vi "BCU诊断标定.vi"(8 "CAN端口":u16(ring), 9 "设备索引号":u16(ring), 10 "CAN卡类型":u32(ring)=21) -> ()   [LabVIEW 2013] (continued)
                                N: w5013 -> [_]
                                tunnel: [""] -> w5019 mode=indexing
                              }
                              n3537 = Multiply(x=u8 3, y=w5014) -> (x*y=w5016:dbl)
                              n3538 = Add(x=w5016, y=u8 23) -> (x+y=w5012:dbl)
                              n3539 = call "表格数据输入-8.6.vi"("行数"=w5012, "列数"=u32 1, "字符串数组"=w5019, "表格引用"=w5020) -> ()  [unwired: 8 in]
                            }
                            frame "保险位置" {
                              n3540 = local read "从板个数"() -> (w5024:dbl)
                              n3541 = control-ref of="项目信息"() -> (w5030:refnum<vi>)
                              n3542 = for {
                                N: 10 -> [_]
                                tunnel: [""] -> w5029 mode=indexing
                              }
                              n3543 = Multiply(x=u8 4, y=w5024) -> (x*y=w5026:dbl)
                              n3544 = Add(x=w5026, y=u8 24) -> (x+y=w5023:dbl)
                              n3545 = call "表格数据输入-8.6.vi"("行数"=w5023, "列数"=u32 1, "字符串数组"=w5029, "表格引用"=w5030) -> ()  [unwired: 8 in]
                            }
                            frame "电池额定实际容量" {
                              w5032 = 0.0 ("值")
                              n3546 = control-ref of="电池实际容量(A)"() -> (w5033:refnum<vi>)
                              n3547 = control-ref of="电池额定容量(A)"() -> (w5034:refnum<vi>)
                              n3548 = property class="DigNum (严格)"(reference=w5033, "Value"=w5032) -> ()  [unwired: 1 in, 2 out]
                              n3549 = property class="DigNum (严格)"(reference=w5034, "Value"=w5032) -> ()  [unwired: 1 in, 2 out]
                            }
                            frame "SOC" {
                              n3550 = control-ref of="SOC(%)"() -> (w5035:refnum<vi>)
                              n3551 = property class="DigNum (严格)"(reference=w5035, "Value"=0.0 ("值")) -> ()  [unwired: 1 in, 2 out]
                            }
                            frame "配置文件版本" {
                              n3552 = control-ref of="配置文件版本"() -> (w5037:refnum<vi>)
                              n3553 = property class="Str"(reference=w5037, "Value"="" ("值")) -> ()  [unwired: 1 in, 2 out]
                            }
                            frame "参数修改记录" {
                              n3554 = control-ref of="使用者"() -> (w5040:refnum<vi>)
                              n3555 = control-ref of="系统时钟"() -> (w5041:refnum<vi>)
                              n3556 = property class="DigNum (严格)"(reference=w5040, "Value"=0.0 ("值")) -> ()  [unwired: 1 in, 2 out]
                              n3557 = property class="Str"(reference=w5041, "Value"="" ("值")) -> ()  [unwired: 1 in, 2 out]
                            }
                            frame "校正时钟" {
                              n3558 = control-ref of="系统时钟"() -> (w5043:refnum<vi>)
                              n3559 = property class="Str"(reference=w5043, "Value"="" ("值")) -> ()  [unwired: 1 in, 2 out]
                            }
                            frame "车牌号" {
                              n3560 = control-ref of="车架(牌)号"() -> (w5045:refnum<vi>)
                              n3561 = property class="Str"(reference=w5045, "Value"="" ("值")) -> ()  [unwired: 1 in, 2 out]
                            }
                            frame "SOH" {
                              n3562 = control-ref of="SOH(%)"() -> (w5048:refnum<vi>)
                              n3563 = property class="DigNum (严格)"(reference=w5048, "Value"=0.0 ("值")) -> ()  [unwired: 1 in, 2 out]
                            }
                            frame "一级故障阀值" {
                              n3564 = local write "一级故障"(T10 {"总电压过高"=0.0, "整组电压不均衡"=0.0, "SOC过高"=0.0, "单体电压过高"=0.0, "总电压过低"=0.0, "温度过高"=0.0, "温度过低"=0.0, "单组电压不均衡"=0.0, "整组温度不均衡"=0.0, "单组温度不均衡"=0.0, "单体电压过低"=0.0, "充电电流过高"=0.0, "放电电流过高"=0.0, "SOC过低"=0.0, "内阻过大"=0.0, "极柱温度过高"=0.0, "SOH过低"=0.0} ("一级故障")) -> ()
                            }
                            frame "二级故障阀值" {
                              n3565 = local write "一级故障 2"(T10 {"总电压过高"=0.0, "整组电压不均衡"=0.0, "SOC过高"=0.0, "单体电压过高"=0.0, "总电压过低"=0.0, "温度过高"=0.0, "温度过低"=0.0, "单组电压不均衡"=0.0, "整组温度不均衡"=0.0, "单组温度不均衡"=0.0, "单体电压过低"=0.0, "充电电流过高"=0.0, "放电电流过高"=0.0, "SOC过低"=0.0, "内阻过大"=0.0, "极柱温度过高"=0.0, "SOH过低"=0.0} ("一级故障")) -> ()
                            }
                            frame "三级故障阀值" {
                              n3566 = local write "一级故障 3"(T10 {"总电压过高"=0.0, "整组电压不均衡"=0.0, "SOC过高"=0.0, "单体电压过高"=0.0, "总电压过低"=0.0, "温度过高"=0.0, "温度过低"=0.0, "单组电压不均衡"=0.0, "整组温度不均衡"=0.0, "单组温度不均衡"=0.0, "单体电压过低"=0.0, "充电电流过高"=0.0, "放电电流过高"=0.0, "SOC过低"=0.0, "内阻过大"=0.0, "极柱温度过高"=0.0, "SOH过低"=0.0} ("一级故障")) -> ()
                            }
                            frame "加热控制参数" {
                              n3567 = local write "加热控制参数"(T11 {"风机开启温度"=0.0, "风机关闭温度"=0.0, "加热开启温度"=0.0, "加热关闭温度"=0.0, "风机开启温差"=0.0, "风机关闭温差"=0.0, "加热关闭温差"=0.0} ("加热控制参数")) -> ()
                            }
                            frame "充电控制参数" {
                              n3568 = local write "一级故障 5"(T12 {"最大允许单体电压"=0.0, "最大允许总电压"=0.0, "最小允许单体电压"=0.0, "最大允许充电电流"=0.0, "最小允许充电电流"=0.0, "最大允许充电温度"=0.0, "最小允许充电温度"=0.0, "电流步长"=0.0} ("一级故障 5")) -> ()
                            }
                            frame "电池信息1" {
                              w5054 = ""
                              w5055 = 0.0 ("电池串联")
                              n3569 = local read "电池信息"() -> (w5057:T13)
                              n3570 = Bundle By Name(cluster=w5057, "电池串联"=w5055, "电池并联"=w5055, "电池包额定容量"=w5055, "电池包额定能量(kWh)"=w5055, "电池包额定总电压"=w5055, "实际容量"=w5055, "电池厂家"=w5054, "电池类型"=w5054, "电池生产日期"=w5054) -> (w5056:T13)
                              n3571 = local write "电池信息"(w5056) -> ()
                            }
                            frame "电池包组号" {
                              n3572 = local read "电池信息"() -> (w5060:T13)
                              n3573 = Bundle By Name(cluster=w5060, "电池包组号"="") -> (w5059:T13)
                              n3574 = local write "电池信息"(w5059) -> ()
                            }
                            frame "充放电安时" {
                              w5061 = 0.0 ("累计充电总安时")
                              n3575 = local read "电池信息"() -> (w5063:T13)
                              n3576 = Bundle By Name(cluster=w5063, "累计充电总安时"=w5061, "累计放电总安时"=w5061) -> (w5062:T13)
                              n3577 = local write "电池信息"(w5062) -> ()
                            }
                            frame "电池充放电次数" {
                              w5064 = 0.0 ("累计充电总安时")
                              n3578 = local read "电池信息"() -> (w5066:T13)
                              n3579 = Bundle By Name(cluster=w5066, "电池充满次数"=w5064, "电池放空次数"=w5064, "电池充电次数"=w5064) -> (w5065:T13)
                              n3580 = local write "电池信息"(w5065) -> ()
                            }
                          }
                        }
                        frame "从板" {
                          n3581 = case shown="\"加热控制参数\"" w5067 {
                            frame "假", Default {
                            }
                            frame "电压起始值" {
                              n3582 = control-ref of="项目信息 2"() -> (w5069:refnum<vi>)
                              n3583 = for {
                                N: 1 -> [_]
                                tunnel: [""] -> w5072 mode=indexing
                              }
                              n3584 = call "表格数据输入-8.6.vi"("行数"=u32 0, "列数"=u32 1, "字符串数组"=w5072, "表格引用"=w5069) -> ()  [unwired: 8 in]
                            }
                            frame "通道电压节数" {
                              n3585 = control-ref of="项目信息 2"() -> (w5074:refnum<vi>)
                              n3586 = for {
                                N: 5 -> [_]
                                tunnel: [""] -> w5078 mode=indexing
                              }
                              n3587 = call "表格数据输入-8.6.vi"("行数"=u32 22, "列数"=u32 1, "字符串数组"=w5078, "表格引用"=w5074) -> ()  [unwired: 8 in]
                            }
                            frame "保险位置" {
                              n3588 = control-ref of="项目信息 2"() -> (w5080:refnum<vi>)
                              n3589 = for {
                                N: 20 -> [_]
                                tunnel: [""] -> w5084 mode=indexing
                              }
                              n3590 = call "表格数据输入-8.6.vi"("行数"=u32 2, "列数"=u32 1, "字符串数组"=w5084, "表格引用"=w5080) -> ()  [unwired: 8 in]
                            }
                            frame "温度起始值" {
                              n3591 = control-ref of="项目信息 2"() -> (w5086:refnum<vi>)
                              n3592 = for {
                                N: 1 -> [_]
                                tunnel: [""] -> w5090 mode=indexing
                              }
                              n3593 = call "表格数据输入-8.6.vi"("行数"=u32 1, "列数"=u32 1, "字符串数组"=w5090, "表格引用"=w5086) -> ()  [unwired: 8 in]
                            }
                            frame "加热控制参数" {
                              n3594 = local write "加热控制参数"(T11 {"风机开启温度"=0.0, "风机关闭温度"=0.0, "加热开启温度"=0.0, "加热关闭温度"=0.0, "风机开启温差"=0.0, "风机关闭温差"=0.0, "加热关闭温差"=0.0} ("加热控制参数")) -> ()
                            }
                            frame "一级故障阀值" {
                              n3595 = local write "一级故障 6"(T15 {"电压过高"=0.0, "电压过低"=0.0, "温度过高"=0.0, "温度过低"=0.0, "电压不均衡(V)"=0.0, "温度不均衡"=0.0, "SOC过低"=0.0} ("一级故障 6")) -> ()
                            }
                            frame "二级故障阀值" {
                              n3596 = local write "一级故障 7"(T15 {"电压过高"=0.0, "电压过低"=0.0, "温度过高"=0.0, "温度过低"=0.0, "电压不均衡(V)"=0.0, "温度不均衡"=0.0, "SOC过低"=0.0} ("一级故障 7")) -> ()
                            }
                            frame "三级故障阀值" {
                              n3597 = local write "一级故障 8"(T15 {"电压过高"=0.0, "电压过低"=0.0, "温度过高"=0.0, "温度过低"=0.0, "电压不均衡(V)"=0.0, "温度不均衡"=0.0, "SOC过低"=0.0} ("一级故障 7")) -> ()
                            }
                            frame "均衡参数" {
                              n3598 = local write "均衡参数"(T17 {"充电结束电压(90%)"=0.0, "充电结束电压(91%)"=0.0, "充电结束电压(92%)"=0.0, "充电结束电压(93%)"=0.0, "充电结束电压(94%)"=0.0, "均衡计算-电压高阀值1级"=0.0, "均衡计算-电压高阀值2级"=0.0, "均衡计算-电压低阀值1级"=0.0, "均衡计算-电压低阀值2级"=0.0, "均衡计算-最低电压阀值"=0.0, "均衡停止-最低电压阀值"=0.0, "均衡计算-电压极差阀值"=0.0, "充电结束电压(95%)"=0.0, "充电结束电压(96%)"=0.0, "充电结束电压(97%)"=0.0, "充电结束电压(98%)"=0.0, "充电结束电压(99%)"=0.0, "充电结束电压(100%)"=0.0} ("均衡参数")) -> ()
                            }
                            frame "均衡阀值" {
                              w5097 = sgl 0.0 ("均衡计算-电压高阀值1级")
                              n3599 = local read "均衡参数"() -> (w5098:T17)
                              n3600 = Bundle By Name(cluster=w5098, "均衡计算-电压高阀值1级"=w5097, "均衡计算-电压高阀值2级"=w5097, "均衡计算-电压低阀值1级"=w5097, "均衡计算-电压低阀值2级"=w5097, "均衡计算-最低电压阀值"=w5097, "均衡停止-最低电压阀值"=w5097, "均衡计算-电压极差阀值"=w5097) -> (w5099:T17)
                              n3601 = local write "均衡参数"(w5099) -> ()
                            }
                            frame "充电结束电压" {
                              w5100 = sgl 0.0 ("均衡计算-电压高阀值1级")
                              n3602 = local read "均衡参数"() -> (w5101:T17)
                              n3603 = Bundle By Name(cluster=w5101, "充电结束电压(90%)"=w5100, "充电结束电压(91%)"=w5100, "充电结束电压(92%)"=w5100, "充电结束电压(93%)"=w5100, "充电结束电压(94%)"=w5100, "充电结束电压(95%)"=w5100, "充电结束电压(96%)"=w5100, "充电结束电压(97%)"=w5100, "充电结束电压(98%)"=w5100, "充电结束电压(99%)"=w5100, "充电结束电压(100%)"=w5100) -> (w5102:T17)
                              n3604 = local write "均衡参数"(w5102) -> ()
                            }
                          }
                        }
                      }
                    }
                    frame #1 {
                      w5103 = FALSE ("流控帧")
                      w5104 = TRUE ("流控帧 2")
                      n3605 = global write "EV05全局变量1.vi" "写入超时"(w5103) -> ()
                      n3606 = global write "EV05全局变量1.vi" "流控帧"(w5103) -> ()
                      n3607 = local write "写?"(w5103) -> ()
                      n3608 = call <vilib>:"Set Busy.vi"("disable click? (T)"=w5103) -> ()  [unwired: 3 in, 8 out]
                      n3609 = local write "消除"(w5104) -> ()
                      n3610 = local write "控制1"(w5104) -> ()
                      n3611 = global write "EV05全局变量1.vi" "流控帧 2"(w5104) -> ()
                    }
                    frame #2 {
                      n3612 = Wait Until Next ms Multiple(millisecond multiple=u32 150 ("毫秒倍数")) -> ()  [unwired: 1 out]
                    }
                    frame #3 {
                      n3613 = local read "设备索引号"() -> (w5111:u16)
                      n3614 = local read "CAN卡类型"() -> (w5112:u32)
                      n3615 = local read "CAN端口"() -> (w5110:u16)
                      n3616 = stacked-sequence {
                        tunnel: w5112 -> [_ w5120]
                        tunnel: w5111 -> [_ w5119]
                        tunnel: w5110 -> [_ w5118]
                        tunnel: w5109 -> [_ w5117]
                        tunnel: w5108 -> [_ w5116]
                        tunnel: w5107 -> [_ w5115]
                        tunnel: w5106 -> [_ w5114]
                        frame #0 {
                        }
                        frame #1 {
                          n3617 = call "多帧发送机制(EV05).vi"("can卡类型"=w5120, "设备索引号"=w5119, "CAN端口"=w5118, "命令"=w5116, "板号"=w5115, "命令序号"=w5117, "输入数据"=w5114) -> ("错误输出"=w5113:errorcluster)  [unwired: 1 in, 11 out]
                          n3618 = call <vilib>:"Clear Errors.vi"("error in (no error)"=w5113) -> ()  [unwired: 6 in, 1 out]
                        }
                      }
                      "命令序号" <- w5109
                    }
                    frame #4 {
                      n3619 = while {
                        tunnel: [w5125] -> w5122
                        tunnel: [w5124] -> w5121
                        i -> [w5128]
                        stop <- w5125 stop-if-true
                        n3620 = local read "强制终止读写标记"() -> (w5123:bool)
                        n3621 = global read "EV05全局变量1.vi" "写入超时"() -> (w5124:bool)
                        n3622 = Greater Or Equal?(x=w5128, y=30) -> (x >= y?=w5126:bool)
                        n3623 = Compound Arithmetic op=OR(w5123, w5124, w5126) -> (w5125:bool)
                        n3624 = Wait Until Next ms Multiple(millisecond multiple=u32 100 ("毫秒倍数")) -> ()  [unwired: 1 out]
                      }
                    }
                    frame #5 {
                      n3625 = call <vilib>:"Unset Busy.vi"() -> ()  [unwired: 11 in, 1 out]
                      n3626 = case shown="假" w5130 {
                        tunnel: w5131 -> [w5134 _]
                        frame False {
                          n3627 = control-ref of="结果"() -> (w5133:refnum<vi>)
                          n3628 = Concatenate Strings(w5134, "     读取失败" ("字符串")) -> (w5136:string)
                          n3629 = Build Array(w5136) -> (w5132:string[])
                          n3630 = call "表格编辑.vi"("新元素/子数组"=w5132, "活动单元格:单元格背景色"=u32 16740749, "MCListbox引用句柄"=w5133) -> ()  [unwired: 9 out]
                        }
                        frame True {
                        }
                      }
                    }
                    frame #6 {
                      n3631 = Increment(x=w5140) -> (x+1=w5139:i32)
                      n3632 = Equal?(x=w5141, y=w5139) -> (x = y?=w5138:bool)
                      n3633 = case shown="真" w5138 {
                        frame False {
                        }
                        frame True {
                          n3634 = control-ref of="结果"() -> (w5143:refnum<vi>)
                          n3635 = Concatenate Strings("读取完成" ("字符串")) -> (w5145:string)
                          n3636 = Build Array(w5145) -> (w5142:string[])
                          n3637 = call "表格编辑.vi"("新元素/子数组"=w5142, "活动单元格:单元格背景色"=u32 21937, "MCListbox引用句柄"=w5143) -> ()  [unwired: 9 out]
                        }
                      }
                    }
                  }
                }
              }
            }
          }
          n3638 = stacked-sequence {
            tunnel: w4795 -> [_]
            frame #0 {
              n3639 = call <vilib>:"Unset Busy.vi"() -> ()  [unwired: 11 in, 1 out]
              n3640 = local write "强制终止读写标记"(FALSE ("强制停止")) -> ()
            }
          }
        }
        frame "全部读取" {
          n3641 = stacked-sequence {
            seq-local: [w5151 _ _] -> [_ _ w5706]
            seq-local: [w5150 _ _] -> [_ _ w5705]
            tunnel: [_ w5342 _] -> w5148
            frame #0 {
              n3642 = local read "主从选择"() -> (w5151:enum32{"主板", "从板"})
              n3643 = local read "路径"() -> (w5152:path)
              n3644 = Empty String/Path?(string/path=w5152) -> (empty?=w5150:bool)
              n3645 = disable-structure shown="禁用" {
                disable-tunnel: w5152 -> [w5155 _]
                disable-tunnel: w5150 -> [w5154 _]
                disable-tunnel: w5151 -> [w5153 _]
                frame Disabled {
                  n3646 = case shown="假" w5154 {
                    tunnel: w5155 -> [w5159 _]
                    tunnel: w5153 -> [w5158 _]
                    frame False {
                      n3647 = control-ref of="结果"() -> (w5156:refnum<vi>)
                      n3648 = call-poly <vilib>:"Read From Spreadsheet File.vi"("file path (dialog if empty)"=w5159) -> ("all rows"=w5157:string[][])  [unwired: 3 in, 7 out]
                      n3649 = case shown="\"主板\", 默认" w5158 {
                        tunnel: w5157 -> [w5161 w5256]
                        tunnel: w5156 -> [w5160 w5255]
                        frame "主板", Default {
                          n3650 = stacked-sequence {
                            tunnel: w5161 -> [w5170 w5194 w5251]
                            tunnel: w5160 -> [w5167 _ w5222]
                            frame #0 {
                              n3651 = Index Array(array=w5170, index (col)=3 ("禁用的索引 (列)")) -> (element=w5184:string[])  [unwired: 1 in]
                              n3652 = Index Array(array=w5170, index (col)=1 ("禁用的索引 (列)")) -> (element=w5190:string[])  [unwired: 1 in]
                              n3653 = Delete From Array(array=w5184, length=4 ("长度"), index=0 ("索引")) -> (deleted portion=w5181:string[], array with subset deleted=w5175:string[])
                              n3654 = Delete From Array(array=w5190, length=1 ("长度"), index=0 ("索引")) -> (deleted portion=w5187:string[], array with subset deleted=w5164:string[])
                              n3655 = Build Array("正在读取主板配置文件...") -> (w5168:string[])
                              n3656 = Index Array(array=w5175) -> (element #1=w5174:string, element #2=w5173:string, element #3=w5172:string, element #4=w5171:string)  [unwired: 4 in]
                              n3657 = for {
                                tunnel: w5181 -> [w5193] mode=indexing
                                tunnel: [w5192] -> w5180 mode=indexing
                                n3658 = Fract/Exp String To Number(string=w5193) -> (number=w5192:dbl)  [unwired: 4 out]
                              }
                              n3659 = Index Array(array=w5187) -> (element=w5186:string)  [unwired: 1 in]
                              n3660 = global write "读配置文件全局.vi" "表格输入"(w5164) -> ()
                              n3661 = call "表格编辑.vi"("新元素/子数组"=w5168, "活动单元格:单元格背景色"=u32 6618880, "MCListbox引用句柄"=w5167) -> ()  [unwired: 9 out]
                              n3662 = Decimal String To Number(string=w5186) -> (number=w5165:i32)  [unwired: 1 in, 2 out]
                              n3663 = global read "读配置文件全局.vi" "项目信息"() -> (w5163:T27)
                              n3664 = Index Array(array=w5180) -> (element #1=w5179:dbl, element #2=w5178:dbl, element #3=w5177:dbl, element #4=w5176:dbl)  [unwired: 4 in]
                              n3665 = global write "读配置文件全局.vi" "从板个数"(w5165) -> ()
                              n3666 = Bundle(cluster=w5163, "电池额定容量"=w5179, "电池实际容量"=w5178, "车牌号"=w5174, "配置文件版本"=w5173, "SOH"=w5176, "SOC"=w5177, "产品编号"=w5172, "系统时钟"=w5171) -> (w5162:T27)  [unwired: 1 out]
                              n3667 = global write "读配置文件全局.vi" "项目信息"(w5162) -> ()
                            }
                            frame #1 {
                              n3668 = Index Array(array=w5194, index (col)=3 ("禁用的索引 (列)")) -> (element=w5212:string[])  [unwired: 1 in]
                              n3669 = Index Array(array=w5194, index (col)=5 ("禁用的索引 (列)")) -> (element=w5206:string[])  [unwired: 1 in]
                              n3670 = for {
                                tunnel: w5206 -> [w5219] mode=indexing
                                tunnel: [w5218] -> w5205 mode=indexing
                                n3671 = Fract/Exp String To Number(string=w5219) -> (number=w5218:dbl)  [unwired: 4 out]
                              }
                              n3672 = Delete From Array(array=w5212, length=17 ("长度"), index=8 ("索引")) -> (deleted portion=w5210:string[])  [unwired: 1 out]
                              n3673 = for {
                                tunnel: w5210 -> [w5221] mode=indexing
                                tunnel: [w5220] -> w5208 mode=indexing
                                n3674 = Fract/Exp String To Number(string=w5221) -> (number=w5220:dbl)  [unwired: 4 out]
                              }
                              n3675 = global write "读配置文件全局.vi" "二级故障"(w5205) -> ()
                              n3676 = global write "读配置文件全局.vi" "一级故障"(w5208) -> ()
                              n3677 = Index Array(array=w5194, index (col)=7 ("禁用的索引 (列)")) -> (element=w5203:string[])  [unwired: 1 in]
                              n3678 = Index Array(array=w5194, index (col)=9 ("禁用的索引 (列)")) -> (element=w5200:string[])  [unwired: 1 in]
                              n3679 = for {
                                tunnel: w5203 -> [w5217] mode=indexing
                                tunnel: [w5216] -> w5202 mode=indexing
                                n3680 = Fract/Exp String To Number(string=w5217) -> (number=w5216:dbl)  [unwired: 4 out]
                              }
                              n3681 = for {
                                tunnel: w5200 -> [w5215] mode=indexing
                                tunnel: [w5214] -> w5199 mode=indexing
                                n3682 = Fract/Exp String To Number(string=w5215) -> (number=w5214:dbl)  [unwired: 4 out]
                              }
                              n3683 = Delete From Array(array=w5199, length=6 ("长度"), index=0 ("索引")) -> (deleted portion=w5196:dbl[], array with subset deleted=w5195:dbl[])
                              n3684 = global write "读配置文件全局.vi" "三级故障"(w5202) -> ()
                              n3685 = global write "读配置文件全局.vi" "加热控制参数"(w5196) -> ()
                              n3686 = global write "读配置文件全局.vi" "充电控制参数"(w5195) -> ()
                            }
                            frame #2 {
                              n3687 = call <vilib>:"Unset Busy.vi"() -> ()  [unwired: 2 in, 10 out]
                              n3688 = Index Array(array=w5251, index (col)=11 ("禁用的索引 (列)")) -> (element=w5248:string[])  [unwired: 1 in]
                              n3689 = Delete From Array(array=w5248, length=6 ("长度"), index=0 ("索引")) -> (deleted portion=w5230:string[], array with subset deleted=w5229:string[])
                              n3690 = for {
                                tunnel: w5229 -> [w5254] mode=indexing
                                tunnel: [w5253] -> w5247 mode=indexing
                                n3691 = Fract/Exp String To Number(string=w5254) -> (number=w5253:dbl)  [unwired: 4 out]
                              }
                              n3692 = Index Array(array=w5230) -> (element #1=w5246:string, element #2=w5245:string, element #3=w5244:string, element #4=w5243:string, element #5=w5242:string, element #6=w5241:string)  [unwired: 6 in]
                              n3693 = Index Array(array=w5247) -> (element #1=w5240:dbl, element #2=w5239:dbl, element #3=w5238:dbl, element #4=w5237:dbl, element #5=w5236:dbl, element #6=w5235:dbl, element #7=w5234:dbl, element #8=w5233:dbl, element #9=w5232:dbl, element #10=w5231:dbl, element #11=w5226:dbl)  [unwired: 11 in]
                              n3694 = global read "读配置文件全局.vi" "电池信息"() -> (w5228:T28)
                              n3695 = Build Array("配置文件读取完成") -> (w5224:string[])
                              n3696 = Bundle(cluster=w5228, "电池串联"=w5240, "电池并联"=w5239, "累计放电总安时"=w5237, "电池包额定容量"=w5236, "电池包额定能量"=w5235, "电池包额定总电压"=w5234, "累计充电总安时"=w5238, "电池充满次数"=w5233, "电池放空次数"=w5232, "电池充电次数"=w5231, "电池生产日期"=w5246, "电池厂家"=w5245, "电池类型"=w5244, "电池包组号"=w5243, "电池包产权标识"=w5242, "电池应用车型"=w5241, "实际容量"=w5226) -> (w5227:T28)
                              n3697 = call "表格编辑.vi"("新元素/子数组"=w5224, "活动单元格:单元格背景色"=u32 6618880, "MCListbox引用句柄"=w5222) -> ()  [unwired: 9 out]
                              n3698 = global write "读配置文件全局.vi" "电池信息"(w5227) -> ()
                            }
                          }
                        }
                        frame "从板" {
                          n3699 = stacked-sequence {
                            tunnel: w5256 -> [w5264 w5292 w5336]
                            tunnel: w5255 -> [w5261 _ w5312]
                            frame #0 {
                              n3700 = Index Array(array=w5264, index (col)=1 ("禁用的索引 (列)")) -> (element=w5274:string[])  [unwired: 1 in]
                              n3701 = Index Array(array=w5264, index (col)=3 ("禁用的索引 (列)")) -> (element=w5268:string[])  [unwired: 1 in]
                              n3702 = Delete From Array(array=w5274, length=1 ("长度"), index=0 ("索引")) -> (deleted portion=w5271:string[], array with subset deleted=w5258:string[])
                              n3703 = Delete From Array(array=w5268, length=6 ("长度"), index=0 ("索引")) -> (deleted portion=w5265:string[])  [unwired: 1 out]
                              n3704 = for {
                                tunnel: w5265 -> [w5277] mode=indexing
                                tunnel: [w5276] -> w5257 mode=indexing
                                i -> [w5278]
                                n3705 = Fract/Exp String To Number(string=w5277, default (0 dbl)=w5278) -> (number=w5276:i32)  [unwired: 3 out]
                              }
                              n3706 = Index Array(array=w5271) -> (element=w5270:string)  [unwired: 1 in]
                              n3707 = global write "读配置文件全局2.vi" "表格"(w5258) -> ()
                              n3708 = Build Array("正在读取从板配置文件...") -> (w5262:string[])
                              n3709 = Decimal String To Number(string=w5270) -> (number=w5259:i32)  [unwired: 1 in, 2 out]
                              n3710 = call "表格编辑.vi"("新元素/子数组"=w5262, "活动单元格:单元格背景色"=u32 6618880, "MCListbox引用句柄"=w5261) -> ()  [unwired: 9 out]
                              n3711 = global write "读配置文件全局2.vi" "加热控制参数"(w5257) -> ()
                              n3712 = global write "读配置文件全局2.vi" "从板板号"(w5259) -> ()
                            }
                            frame #1 {
                              n3713 = Index Array(array=w5292, index (col)=3 ("禁用的索引 (列)")) -> (element=w5282:string[])  [unwired: 1 in]
                              n3714 = Array Subset(array=w5282, index=6 ("索引"), length=7 ("长度")) -> (w5289:string[])
                              n3715 = Array Subset(array=w5282, index=13 ("索引"), length=7 ("长度")) -> (w5288:string[])
                              n3716 = Array Subset(array=w5282, index=20 ("索引"), length=7 ("长度")) -> (w5283:string[])
                              n3717 = for {
                                tunnel: w5289 -> [w5299] mode=indexing
                                tunnel: [w5298] -> w5279 mode=indexing
                                n3718 = Fract/Exp String To Number(string=w5299) -> (number=w5298:dbl)  [unwired: 4 out]
                              }
                              n3719 = for {
                                tunnel: w5288 -> [w5297] mode=indexing
                                tunnel: [w5296] -> w5280 mode=indexing
                                n3720 = Fract/Exp String To Number(string=w5297) -> (number=w5296:dbl)  [unwired: 4 out]
                              }
                              n3721 = for {
                                tunnel: w5283 -> [w5295] mode=indexing
                                tunnel: [w5294] -> w5281 mode=indexing
                                n3722 = Fract/Exp String To Number(string=w5295) -> (number=w5294:dbl)  [unwired: 4 out]
                              }
                              n3723 = global write "读配置文件全局2.vi" "一级故障阀值"(w5279) -> ()
                              n3724 = global write "读配置文件全局2.vi" "二级故障阀值"(w5280) -> ()
                              n3725 = global write "读配置文件全局2.vi" "三级故障阀值"(w5281) -> ()
                            }
                            frame #2 {
                              n3726 = Index Array(array=w5336, index (col)=5 ("禁用的索引 (列)")) -> (element=w5334:string[])  [unwired: 1 in]
                              n3727 = Delete From Array(array=w5334, length=1 ("长度"), index=16 ("索引")) -> (deleted portion=w5330:string[], array with subset deleted=w5331:string[])
                              n3728 = for {
                                tunnel: w5331 -> [w5339] mode=indexing
                                tunnel: [w5338] -> w5335 mode=indexing
                                n3729 = Fract/Exp String To Number(string=w5339) -> (number=w5338:dbl)  [unwired: 4 out]
                              }
                              n3730 = Index Array(array=w5335) -> (element #1=w5329:dbl, element #2=w5328:dbl, element #3=w5327:dbl, element #4=w5326:dbl, element #5=w5325:dbl, element #6=w5324:dbl, element #7=w5323:dbl, element #8=w5322:dbl, element #9=w5321:dbl, element #10=w5320:dbl, element #11=w5319:dbl, element #12=w5310:dbl, element #13=w5318:dbl, element #14=w5317:dbl, element #15=w5316:dbl, element #16=w5315:dbl, element #17=w5308:dbl, element #18=w5307:dbl, element #19=w5306:dbl, element #20=w5305:dbl, element #21=w5304:dbl, element #22=w5303:dbl)  [unwired: 22 in]
                              n3731 = Build Array("配置文件读取完成") -> (w5313:string[])
                              n3732 = Index Array(array=w5330, index=22 ("索引")) -> (element=w5309:string)
                              n3733 = global read "读配置文件全局2.vi" "电池组信息"() -> (w5301:T29)
                              n3734 = call "表格编辑.vi"("新元素/子数组"=w5313, "活动单元格:单元格背景色"=u32 6618880, "MCListbox引用句柄"=w5312) -> ()  [unwired: 9 out]
                              n3735 = Bundle(cluster=w5301, "电池类型"=w5329, "电池厂家"=w5328, "电池地区"=w5327, "电池组序号"=w5326, "电池包串联数"=w5325, "电池包并联数"=w5324, "电池包安时数"=w5323, "电池包序号"=w5322, "充电次数"=w5321, "充满电时间"=w5320, "放空时间"=w5319, "车牌号"=w5309, "最大允许单体电压"=w5310, "最大允许总电压"=w5318, "最大允许温度"=w5317, "最小允许温度"=w5316, "最大允许充电电流"=w5315, "最小允许充电电流"=w5308, "最小允许单体电压"=w5307, "电流步长"=w5306, "SOC"=w5305, "充电总安时"=w5304, "放电总这时"=w5303) -> (w5300:T29)
                              n3736 = call <vilib>:"Unset Busy.vi"() -> ()  [unwired: 2 in, 10 out]
                              n3737 = global write "读配置文件全局2.vi" "电池组信息"(w5300) -> ()
                            }
                          }
                        }
                      }
                    }
                    frame True {
                    }
                  }
                }
                frame Enabled {
                }
              }
              n3738 = case shown="\"从板\"" w5151 {
                frame "主板", Default {
                  w5340 = FALSE
                  n3739 = global write "读配置文件全局.vi" "SOC判定"(w5340) -> ()
                  n3740 = global write "读配置文件全局.vi" "SOH判定"(w5340) -> ()
                  n3741 = global write "读配置文件全局.vi" "车牌号判定"(w5340) -> ()
                  n3742 = global write "读配置文件全局.vi" "电池信息1判定"(w5340) -> ()
                  n3743 = global write "读配置文件全局.vi" "保险位置判定"(w5340) -> ()
                  n3744 = global write "读配置文件全局.vi" "产品编号判定"(w5340) -> ()
                  n3745 = global write "读配置文件全局.vi" "充放电安时判定"(w5340) -> ()
                  n3746 = global write "读配置文件全局.vi" "从板个数判定"(w5340) -> ()
                  n3747 = global write "读配置文件全局.vi" "电池包组号判定"(w5340) -> ()
                  n3748 = global write "读配置文件全局.vi" "电压个数判定"(w5340) -> ()
                  n3749 = global write "读配置文件全局.vi" "电压起始值判定"(w5340) -> ()
                  n3750 = global write "读配置文件全局.vi" "二级故障判定"(w5340) -> ()
                  n3751 = global write "读配置文件全局.vi" "三级故障判定"(w5340) -> ()
                  n3752 = global write "读配置文件全局.vi" "通道电压数判定"(w5340) -> ()
                  n3753 = global write "读配置文件全局.vi" "温度个数判定"(w5340) -> ()
                  n3754 = global write "读配置文件全局.vi" "一级故障判定"(w5340) -> ()
                  n3755 = global write "读配置文件全局.vi" "温度起始值判定"(w5340) -> ()
                  n3756 = global write "读配置文件全局.vi" "充电控制参数判定"(w5340) -> ()
                  n3757 = global write "读配置文件全局.vi" "电池充放电次数判定"(w5340) -> ()
                  n3758 = global write "读配置文件全局.vi" "加热控制参数判定"(w5340) -> ()
                  n3759 = global write "读配置文件全局.vi" "配置文件版本判定"(w5340) -> ()
                  n3760 = global write "读配置文件全局.vi" "电池额定实际容量判定"(w5340) -> ()
                }
                frame "从板" {
                  w5341 = FALSE
                  n3761 = disable-structure shown="禁用" {
                    frame Disabled {
                      n3762 = global read "读配置文件全局2.vi" "充电次数时间判定"() -> ()  [unwired: 1 in]
                      n3763 = global read "读配置文件全局2.vi" "电池包信息1判定"() -> ()  [unwired: 1 in]
                      n3764 = global read "读配置文件全局2.vi" "电池包序号判定"() -> ()  [unwired: 1 in]
                      n3765 = global read "读配置文件全局2.vi" "充放电安时判定"() -> ()  [unwired: 1 in]
                      n3766 = global read "读配置文件全局2.vi" "车牌号判定"() -> ()  [unwired: 1 in]
                      n3767 = global read "读配置文件全局2.vi" "充电参数判定"() -> ()  [unwired: 1 in]
                      n3768 = global read "读配置文件全局2.vi" "保险位置判定"() -> ()  [unwired: 1 in]
                    }
                    frame Enabled {
                    }
                  }
                  n3769 = global write "读配置文件全局2.vi" "从板号判定"(w5341) -> ()
                  n3770 = global write "读配置文件全局2.vi" "通道电压判定"(w5341) -> ()
                  n3771 = global write "读配置文件全局2.vi" "保险位置判定"(w5341) -> ()
                  n3772 = global write "读配置文件全局2.vi" "二级故障判定"(w5341) -> ()
                  n3773 = global write "读配置文件全局2.vi" "三级故障判定"(w5341) -> ()
                  n3774 = global write "读配置文件全局2.vi" "一级故障判定"(w5341) -> ()
                  n3775 = global write "读配置文件全局2.vi" "电压起始值判定"(w5341) -> ()
                  n3776 = global write "读配置文件全局2.vi" "温度起始值判定"(w5341) -> ()
                }
              }
            }
            frame #1 {
              (unwired) "均衡参数"
              # "去掉加热控制信息 20140106"
              n3777 = local read "主从选择"() -> (w5345:enum32{"主板", "从板"})
              n3778 = case shown="\"主板\", 默认" w5345 {
                tunnel: [string[] ["项目信息", "一级故障阀值", "二级故障阀值", "三级故障阀值", "加热控制信息", "充电控制信息", "电池信息"] string[] ["从板信息", "一级故障阀值", "二级故障阀值", "三级故障阀值"]] -> w5344
                frame "主板", Default {
                }
                frame "从板" {
                }
              }
              n3779 = Array Size(array=w5344) -> (size(s)=w5343:i32)
              n3780 = for {
                tunnel: w5344 -> [w5361] mode=indexing
                tunnel: w5345 -> [w5349]
                tunnel: w5343 -> [w5353]
                tunnel: [w5348] -> w5342
                i -> [w5350]
                n3781 = case shown="\"主板\", 默认" w5349 {
                  tunnel: [w5657 w5685] -> w5355
                  tunnel: [w5656 w5686] -> w5356
                  tunnel: w5361 -> [w5653 w5682]
                  tunnel: [u8 0 ("板号") w5683] -> w5360
                  tunnel: [u8 0 ("板号") u8 0 ("板号")] -> w5359
                  tunnel: [w5652 w5681] -> w5357
                  frame "主板", Default {
                    n3782 = case shown="\"项目信息\"" w5653 {
                      tunnel: [_ u8[] [1, 2, 3, 4, 5, 6, 13, 8, 7, 9, 10, 11, 12] u8[] [1] u8[] [2] u8[] [3] u8[] [1] u8[] [2] u8[] [1, 2, 3] u8[] [1, 2, 3, 4]] -> w5657
                      tunnel: [_ u8 128 ("命令") u8 129 ("命令") u8 129 ("命令") u8 129 ("命令") u8 130 ("命令") u8 130 ("命令") u8 131 ("命令") u8 132 ("命令")] -> w5656
                      tunnel: [_ string[] ["产品编号", "电压个数", "通道电压数", "电压起始值", "温度个数", "温度起始值", "保险位置", "电池额定实际容量", "SOC", "配置文件版本", "参数修改记录", "车牌号", "SOH"] string[] ["一级故障阀值"] string[] ["二级故障阀值"] string[] ["三级故障阀值"] string[] ["加热控制参数"] string[] ["充电控制参数"] _ string[] ["电池信息1", "电池包组号", "充放电安时", "电池充放电次数"]] -> w5652
                      frame "假", Default {
                      }
                      frame "项目信息" {
                      }
                      frame "一级故障阀值" {
                      }
                      frame "二级故障阀值" {
                      }
                      frame "三级故障阀值" {
                      }
                      frame "加热控制信息" {
                      }
                      frame "充电控制信息" {
                      }
                      frame "历史信息" {
                      }
                      frame "电池信息" {
                      }
                    }
                  }
                  frame "从板" {
                    n3783 = case shown="\"从板信息\"" w5682 {
                      tunnel: [_ u8 0 ("命令") u8 2 ("命令") u8 2 ("命令") u8 2 ("命令") u8 3 ("命令") u8 6 ("命令")] -> w5686
                      tunnel: [_ u8[] [6, 1, 2, 3, 4, 5] u8[] [1] u8[] [2] u8[] [3] u8[] [1, 2, 3, 4, 5, 6, 7] u8[] [1, 2]] -> w5685
                      tunnel: [_ string[] ["从板号", "电压起始值", "通道电压节数", "保险位置", "温度起始值", "加热控制参数"] string[] ["一级故障阀值"] string[] ["二级故障阀值"] string[] ["三级故障阀值"] string[] ["电池包信息1", "电池包序号", "充放电安时", "充电次数时间", "SOC", "车牌号", "充电参数"] string[] ["均衡阀值", "充电结束电压"]] -> w5681
                      frame "假", Default {
                      }
                      frame "从板信息" {
                      }
                      frame "一级故障阀值" {
                      }
                      frame "二级故障阀值" {
                      }
                      frame "三级故障阀值" {
                      }
                      frame "快换参数" {
                      }
                      frame "均衡参数" {
                      }
                    }
                    n3784 = local read "从板号"() -> (w5683:u8)
                  }
                }
                n3785 = Increment(x=w5350) -> (x+1=w5352:i32)
                n3786 = Equal?(x=w5353, y=w5352) -> (x = y?=w5351:bool)
                n3787 = case shown="\"从板\"" w5349 {
                  tunnel: w5350 -> [w5623 w5637]
                  frame "主板", Default {
                    n3788 = case shown="0, 默认" w5623 {
                      tunnel: [T8."项目信息" ("主从板") T8."一级故障阀值" ("主从板") T8."二级故障阀值" ("主从板") T8."三级故障阀值" ("主从板") T8."控制参数" ("主从板") T8."电池信息" ("主从板")] -> w5622
                      frame 0, Default {
                        n3789 = local write "1"(TRUE ("1")) -> ()
                      }
                      frame 1 {
                        n3790 = local write "1 2"(TRUE ("1 2")) -> ()
                      }
                      frame 2 {
                        n3791 = local write "1 3"(TRUE ("1 3")) -> ()
                      }
                      frame 3 {
                        n3792 = local write "1 4"(TRUE ("1 4")) -> ()
                      }
                      frame 4, 5 {
                        n3793 = local write "1 5"(TRUE ("1 5")) -> ()
                      }
                      frame 6 {
                        n3794 = local write "1 11"(TRUE ("1 11")) -> ()
                      }
                    }
                    n3795 = local write "主板2"(w5622) -> ()
                  }
                  frame "从板" {
                    n3796 = case shown="4" w5637 {
                      tunnel: [T21."从板信息" ("等级 2") T21."从板信息" ("等级 2") T21."一级故障阀值" ("等级 2") T21."二级故障阀值" ("等级 2") T21."三级故障阀值" ("等级 2") T21."快换参数" ("等级 2") T14."均衡参数" ("等级 2")] -> w5636
                      frame 99, Default {
                        n3797 = local write "1 6"(TRUE ("1 6")) -> ()
                      }
                      frame 0 {
                        n3798 = local write "1 6"(TRUE ("1 6")) -> ()
                      }
                      frame 1 {
                        n3799 = local write "1 7"(TRUE ("1 7")) -> ()
                      }
                      frame 2 {
                        n3800 = local write "1 8"(TRUE ("1 8")) -> ()
                      }
                      frame 3 {
                        n3801 = local write "1 9"(TRUE ("1 9")) -> ()
                      }
                      frame 5 {
                        n3802 = local write "1 10"(TRUE ("1 10")) -> ()
                      }
                      frame 4 {
                        n3803 = local write "1 12"(TRUE ("1 10")) -> ()
                      }
                    }
                    n3804 = local write "等级 2"(w5636) -> ()
                  }
                }
                n3805 = Array Size(array=w5355) -> (size(s)=w5354:i32)
                n3806 = local write "命令"(w5356) -> ()
                n3807 = Build Array(w5359) -> (w5358:u8[])
                n3808 = while {
                  tunnel: w5356 -> [w5393]
                  tunnel: w5360 -> [w5392]
                  tunnel: w5358 -> [w5391]
                  tunnel: w5354 -> [w5387]
                  tunnel: w5351 -> [w5390]
                  tunnel: w5349 -> [w5384]
                  tunnel: [w5383] -> w5348
                  shift-right: [w5382] -> _
                  shift-left: w5357 -> [w5363]
                  shift-right: [w5373] -> _
                  shift-left: w5355 -> [w5362]
                  i -> [w5388]
                  stop <- w5383 stop-if-true
                  n3809 = local read "强制终止读写标记"() -> (w5379:bool)
                  n3810 = Array Size(array=w5363) -> (size(s)=w5381:i32)
                  n3811 = Increment(x=w5388) -> (x+1=w5389:i32)
                  n3812 = Greater Than 0?(x=w5381) -> (x > 0?=w5380:bool)
                  n3813 = Equal?(x=w5387, y=w5389) -> (x = y?=w5385:bool)
                  n3814 = Not(x=w5379) -> (.not. x?=w5378:bool)
                  n3815 = And(x=w5378, y=w5380) -> (x .and. y?=w5377:bool)
                  n3816 = Delete From Array(array=w5363, length=1 ("长度"), index=0 ("索引")) -> (deleted portion=w5369:string[], array with subset deleted=w5374:string[])
                  n3817 = Index Array(array=w5369, index=0 ("索引")) -> (element=w5367:string)
                  n3818 = Delete From Array(array=w5362, length=1 ("长度"), index=0 ("索引")) -> (deleted portion=w5365:u8[], array with subset deleted=w5370:u8[])
                  n3819 = Index Array(array=w5365, index=0 ("索引")) -> (element=w5364:u8)
                  n3820 = case shown="真" w5377 {
                    tunnel: w5393 -> [_ w5409]
                    tunnel: w5364 -> [_ w5408]
                    tunnel: w5392 -> [_ w5407]
                    tunnel: w5391 -> [_ w5406]
                    tunnel: w5367 -> [_ w5405]
                    tunnel: w5390 -> [_ w5404]
                    tunnel: w5385 -> [_ w5403]
                    tunnel: w5384 -> [_ w5402]
                    tunnel: [string[] [] w5398] -> w5382
                    tunnel: w5374 -> [_ w5401]
                    tunnel: [u8[] [] w5396] -> w5373
                    tunnel: w5370 -> [_ w5400]
                    tunnel: w5363 -> [_ w5399]
                    tunnel: w5362 -> [_ w5397]
                    frame False {
                    }
                    frame True {
                      n3821 = while {
                        tunnel: w5409 -> [w5425]
                        tunnel: w5408 -> [w5424]
                        tunnel: w5407 -> [w5423]
                        tunnel: w5406 -> [w5422]
                        tunnel: w5405 -> [w5420]
                        tunnel: w5404 -> [w5419]
                        tunnel: w5403 -> [w5418]
                        tunnel: w5402 -> [w5417]
                        tunnel: w5401 -> [w5413]
                        tunnel: w5400 -> [w5411]
                        tunnel: w5399 -> [w5414]
                        tunnel: [w5415] -> w5398
                        tunnel: w5397 -> [w5412]
                        tunnel: [w5410] -> w5396
                        i -> [w5416]
                        stop <- w5421 stop-if-true
                        n3822 = stacked-sequence {
                          seq-local: [_ _ _ _ w5572 _ _] -> [_ _ _ _ _ w5588 _]
                          tunnel: w5425 -> [_ _ _ w5564 _ _ _]
                          tunnel: w5424 -> [_ _ _ w5563 _ _ _]
                          tunnel: w5423 -> [_ _ _ w5562 _ _ _]
                          tunnel: w5422 -> [_ _ _ w5561 _ _ _]
                          tunnel: [_ _ _ _ w5573 _ _] -> w5421
                          tunnel: w5420 -> [w5427 _ _ _ _ w5587 _]
                          tunnel: w5419 -> [_ _ _ _ _ _ w5615]
                          tunnel: w5418 -> [_ _ _ _ _ _ w5613]
                          tunnel: w5417 -> [w5426 _ _ _ _ _ _]
                          tunnel: w5416 -> [_ _ _ _ _ _ _]
                          tunnel: [_ _ _ _ _ w5586 _] -> w5415
                          tunnel: w5414 -> [_ _ _ _ _ w5585 _]
                          tunnel: w5413 -> [_ _ _ _ _ w5584 _]
                          tunnel: w5412 -> [_ _ _ _ _ w5583 _]
                          tunnel: w5411 -> [_ _ _ _ _ w5582 _]
                          tunnel: [_ _ _ _ _ w5581 _] -> w5410
                          frame #0 {
                            n3823 = case shown="\"主板\", 默认" w5426 {
                              tunnel: w5427 -> [w5428 w5519]
                              frame "主板", Default {
                                n3824 = case shown="\"电池包组号\"" w5428 {
                                frame "假", Default {
                                }
                                frame "产品编号" {
                                n3825 = control-ref of="产品编号"() -> (w5430:refnum<vi>)
                                n3826 = property class="Str"(reference=w5430, "Value"="") -> ()  [unwired: 1 in, 2 out]
                                }
                                frame "电压个数" {
                                n3827 = local read "从板个数"() -> (w5431:dbl)
                                n3828 = control-ref of="项目信息"() -> (w5435:refnum<vi>)
                                n3829 = for {
                                N: w5431 -> [_]
                                tunnel: [""] -> w5434 mode=indexing
                                }
                                n3830 = call "表格数据输入-8.6.vi"("行数"=u32 0, "列数"=u32 1, "字符串数组"=w5434, "表格引用"=w5435) -> ()  [unwired: 8 in]
                                }
                                frame "通道电压数" {
                                n3831 = disable-structure shown="禁用" {
                                frame Disabled {
                                n3832 = control-ref of="项目信息"() -> (w5441:refnum<vi>)
                                n3833 = for {
                                N: 20 -> [_]
                                tunnel: [""] -> w5440 mode=indexing
                                }
                                n3834 = local read "从板个数"() -> (w5442:dbl)
                                n3835 = Increment(x=w5442) -> (x+1=w5438:dbl)
                                n3836 = call "表格数据输入-8.6.vi"("行数"=w5438, "列数"=u32 1, "字符串数组"=w5440, "表格引用"=w5441) -> ()  [unwired: 8 in]
                                }
                                frame Enabled {
                                }
                                }
                                }
                                frame "电压起始值" {
                                n3837 = disable-structure shown="禁用" {
                                frame Disabled {
                                n3838 = local read "从板个数"() -> (w5446:dbl)
                                n3839 = Increment(x=w5446) -> (x+1=w5445:dbl)
                                n3840 = control-ref of="项目信息"() -> (w5452:refnum<vi>)
                                n3841 = for {
                                N: w5445 -> [_]
                                tunnel: [""] -> w5451 mode=indexing
                                }
                                n3842 = Multiply(x=u8 1, y=w5446) -> (x*y=w5448:dbl)
                                n3843 = Add(x=w5448, y=u8 21) -> (x+y=w5444:dbl)
                                n3844 = call "表格数据输入-8.6.vi"("行数"=w5444, "列数"=u32 1, "字符串数组"=w5451, "表格引用"=w5452) -> ()  [unwired: 8 in]
                                }
                                frame Enabled {
                                }
                                }
                                }
                                frame "温度个数" {
                                n3845 = local read "从板个数"() -> (w5456:dbl)
                                n3846 = Increment(x=w5456) -> (x+1=w5455:dbl)
                                n3847 = control-ref of="项目信息"() -> (w5462:refnum<vi>)
                                n3848 = for {
                                N: w5455 -> [_]
                                tunnel: [""] -> w5461 mode=indexing
                                }
                                n3849 = Multiply(x=u8 2, y=w5456) -> (x*y=w5458:dbl)
                                n3850 = Add(x=w5458, y=u8 22) -> (x+y=w5454:dbl)
                                n3851 = call "表格数据输入-8.6.vi"("行数"=w5454, "列数"=u32 1, "字符串数组"=w5461, "表格引用"=w5462) -> ()  [unwired: 8 in]
                                }
                                frame "温度起始值" {
                                n3852 = disable-structure shown="禁用" {
                                frame Disabled {
                                n3853 = local read "从板个数"() -> (w5466:dbl)
                                n3854 = Increment(x=w5466) -> (x+1=w5465:dbl)
                                n3855 = control-ref of="项目信息"() -> (w5472:refnum<vi>)
                                n3856 = for {
                                N: w5465 -> [_]
                                tunnel: [""] -> w5471 mode=indexing
                                }
                                n3857 = Multiply(x=u8 3, y=w5466) -> (x*y=w5468:dbl)
                                n3858 = Add(x=w5468, y=u8 23) -> (x+y=w5464:dbl)
                                n3859 = call "表格数据输入-8.6.vi"("行数"=w5464, "列数"=u32 1, "字符串数组"=w5471, "表格引用"=w5472) -> ()  [unwired: 8 in]
                                }
                                frame Enabled {
                                }
                                }
                                }
                                frame "保险位置" {
                                n3860 = local read "从板个数"() -> (w5476:dbl)
                                n3861 = control-ref of="项目信息"() -> (w5482:refnum<vi>)
                                n3862 = for {
                                N: 10 -> [_]
                                tunnel: [""] -> w5481 mode=indexing
                                }
                                n3863 = Multiply(x=u8 4, y=w5476) -> (x*y=w5478:dbl)
                                n3864 = Add(x=w5478, y=u8 24) -> (x+y=w5475:dbl)
                                n3865 = call "表格数据输入-8.6.vi"("行数"=w5475, "列数"=u32 1, "字符串数组"=w5481, "表格引用"=w5482) -> ()  [unwired: 8 in]
                                }
                                frame "电池额定实际容量" {
                                w5484 = 0.0 ("值")
                                n3866 = control-ref of="电池实际容量(A)"() -> (w5485:refnum<vi>)
                                n3867 = control-ref of="电池额定容量(A)"() -> (w5486:refnum<vi>)
                                n3868 = property class="DigNum (严格)"(reference=w5485, "Value"=w5484) -> ()  [unwired: 1 in, 2 out]
                                n3869 = property class="DigNum (严格)"(reference=w5486, "Value"=w5484) -> ()  [unwired: 1 in, 2 out]
                                }
                                frame "SOC" {
                                n3870 = control-ref of="SOC(%)"() -> (w5487:refnum<vi>)
                                n3871 = property class="DigNum (严格)"(reference=w5487, "Value"=0.0 ("值")) -> ()  [unwired: 1 in, 2 out]
                                }
                                frame "配置文件版本" {
                                n3872 = control-ref of="配置文件版本"() -> (w5489:refnum<vi>)
                                n3873 = property class="Str"(reference=w5489, "Value"="" ("值")) -> ()  [unwired: 1 in, 2 out]
                                }
                                frame "参数修改记录" {
                                n3874 = control-ref of="使用者"() -> (w5492:refnum<vi>)
                                n3875 = control-ref of="系统时钟"() -> (w5493:refnum<vi>)
                                n3876 = property class="DigNum (严格)"(reference=w5492, "Value"=0.0 ("值")) -> ()  [unwired: 1 in, 2 out]
                                n3877 = property class="Str"(reference=w5493, "Value"="" ("值")) -> ()  [unwired: 1 in, 2 out]
                                }
                                frame "校正时钟" {
                                n3878 = control-ref of="系统时钟"() -> (w5495:refnum<vi>)
                                n3879 = property class="Str"(reference=w5495, "Value"="" ("值")) -> ()  [unwired: 1 in, 2 out]
                                }
                                frame "车牌号" {
                                n3880 = control-ref of="车架(牌)号"() -> (w5497:refnum<vi>)
                                n3881 = property class="Str"(reference=w5497, "Value"="" ("值")) -> ()  [unwired: 1 in, 2 out]
                                }
                                frame "SOH" {
                                n3882 = control-ref of="SOH(%)"() -> (w5500:refnum<vi>)
                                n3883 = property class="DigNum (严格)"(reference=w5500, "Value"=0.0 ("值")) -> ()  [unwired: 1 in, 2 out]
                                }
                                frame "一级故障阀值" {
                                n3884 = local write "一级故障"(T10 {"总电压过高"=0.0, "整组电压不均衡"=0.0, "SOC过高"=0.0, "单体电压过高"=0.0, "总电压过低"=0.0, "温度过高"=0.0, "温度过低"=0.0, "单组电压不均衡"=0.0, "整组温度不均衡"=0.0, "单组温度不均衡"=0.0, "单体电压过低"=0.0, "充电电流过高"=0.0, "放电电流过高"=0.0, "SOC过低"=0.0, "内阻过大"=0.0, "极柱温度过高"=0.0, "SOH过低"=0.0} ("一级故障")) -> ()
                                }
                                frame "二级故障阀值" {
